vi "set_op_no.vi"(8 "error in (no error)":errorcluster, 10 "op_no":T1, 11 "SsaId in":refnum<class "SsaId.lvclass">) -> (0 "error out":errorcluster, 3 "SsaId out":refnum<class "SsaId.lvclass">)   [LabVIEW 2020, in "mlir.lvlib" / "SsaId.lvclass"]
uses:
  SsaId.lvclass
  op_no.ctl
  SsaId.lvclass/SsaId.ctl
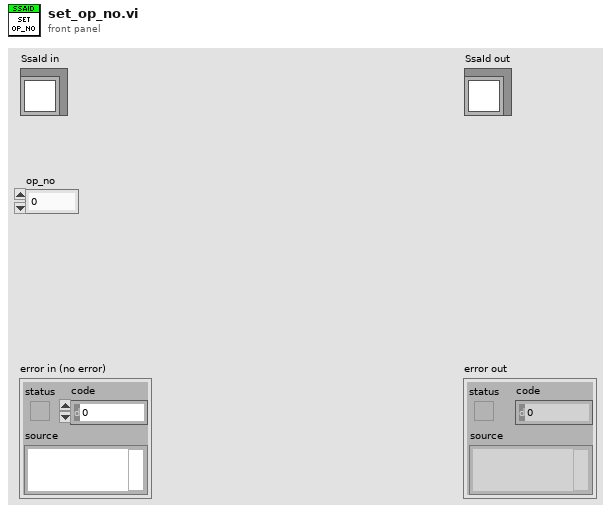
[diagram p1: front panel]
types:
  T1 = typedef "mlir.lvlib/SsaId.lvclass/op_no.ctl" = u32
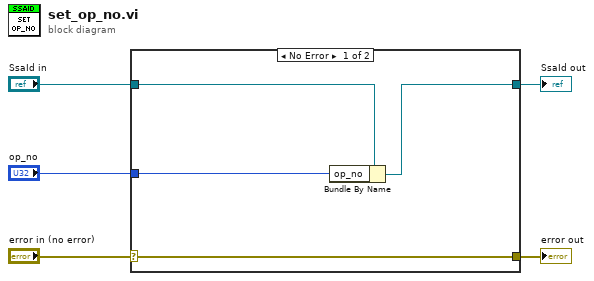
[diagram p0: block diagram]
diagram:
  n1 = case shown="No Error" "error in (no error)" {
    selector: "error in (no error)" -> [w9 w10]
    tunnel: [w9 w10] -> w4
    tunnel: [w7 w11] -> w2
    tunnel: "SsaId in" -> [w8 w11]
    tunnel: "op_no" -> [w6 _]
    frame No Error {
      n2 = Bundle By Name(cluster=w8, "op_no"=w6) -> (w7:refnum<class "SsaId.lvclass">)
    }
    frame Error {
    }
  }
  "error out" <- w4
  "SsaId out" <- w2
